vi "Least Pth Norm IIR Filter Design.vi"() -> ()   [LabVIEW 2023]
doc: "Demonstrates how to use the DFD Least Pth Norm Design VI to design advanced infinite impulse response (IIR) filters. You can learn how to configure the controls to obtain the ideal frequency response of the filter you want to design.\n\nComplete the following steps to use this VI.\n1) Run the VI.\n2) Select one example filter in the <B>Examples</B> list. This VI provides pre-defined filter specifications for each example filter.\n3) View the <B>Specifications</B> page to study the corresponding settings that describe the ideal frequency response.\n4) Observe the magnitude response and the pole-zero plot to view the characteristics of the designed filter.\n5) Click the <B>STOP</B> button to stop this VI."
uses:
  <vilib>/addons/Digital Filter Design/_Objects.llb/DFD Pole-Zero Plot.ctl
  <vilib>/addons/Digital Filter Design/_LpNorm.llb/dfd_Lp Norm Filter Type.ctl
  <vilib>/addons/Digital Filter Design/_Objects.llb/DFD Filter Obj.ctl
  <vilib>/addons/Digital Filter Design/_Objects.llb/DFD Filter Coef.ctl
  <vilib>/addons/Digital Filter Design/_Objects.llb/DFD Filter Structure Type Selector.ctl
  <vilib>/addons/Digital Filter Design/_Objects.llb/dfd_Internal Quantization Settings.ctl
  <vilib>/addons/Digital Filter Design/_Objects.llb/dfd_Internal Quantization Srcs.ctl
  <vilib>/addons/Digital Filter Design/_Objects.llb/DFD Coef Norm Type.ctl
  <vilib>/addons/Digital Filter Design/_Objects.llb/DFD Phase Setting.ctl
  <vilib>/addons/Digital Filter Design/Design.llb/DFD Least Pth Norm Design by IRLS.vi
  <vilib>/addons/Digital Filter Design/Analysis.llb/DFD Plot Freq Response (Linear-Spaced).vi
  <vilib>/addons/Digital Filter Design/NI_DigFilterLicensed.lvlib
panel:
  in  "filter out":T1={"mSRate_Fs"=1.0, "mSRate_Version"="1.0", "mSRate_Comments"="", "mSRate_OrgCoef"={"type"=enum."Undefined", "gain"=1.0, "coef a (k)"=[], "coef b (v)"=[]}, "mSRate_CurCoef"={"type"=enum."Undefined", "gain"=1.0, "coef a (k)"=[], "coef b (v)"=[]}, "mSRate_Quantized?"=FALSE, "mSRate_QCoef"={"type"=enum."Undefined", "gain"=1.0, "coef a (k)"=[], "coef b (v)"=[]}, "mSRate_QSettings"=[], "mSRate_Order"=0, "mSRate_Scaling"={"mSRate_ScaleByPowerOf2?"=FALSE, "mSRate_ScaleType"=enum."No Norm"}} {"mSRate_QSettings"."source" items=["Coef a/k"=0, "Coef b/v"=7, "Input"=1, "Output"=2, "Multiplicand"=3, "Product"=4, "Sum"=5, "Delay"=6, "Gain"=8]}
  out "Status Str":string="Idle"
  out "Status LED":bool
  in  "Graph":T7(tab)
  in  "dB on?":bool=TRUE
  out "Magnitude Response":cluster{"f0":dbl, "df":dbl, "values":dbl[]}[](graph)
  in  "phase view":T8
  out "Phase Response":cluster{"f0":dbl, "df":dbl, "values":dbl[]}[](graph)
  out "Group Delay":cluster{"f0":dbl, "df":dbl, "values":dbl[]}[](graph)
  out "Z-Plane":T9
  in  "stop":bool
  in  "Selector":enum32{"Examples", "Specifications"}(tab)
  out "Description":string
  in  "Example List":i32(listbox)
  in  "Apply":bool
  in  "p":i32=128
  in  "Group Delay":dbl=5.0
  in  "Band Specifications":T10(array[cluster])=[{"frequency point"=[{"frequency"=0.0, "magnitude"=1.0, "weight"=1.0, "phase"=0.0}, {"frequency"=0.2, "magnitude"=1.0, "weight"=1.0, "phase"=0.0}]}, {"frequency point"=[{"frequency"=0.3, "magnitude"=0.0, "weight"=1.0, "phase"=0.0}, {"frequency"=0.5, "magnitude"=0.0, "weight"=1.0, "phase"=0.0}]}] {"frequency point"."weight" format="%.2f"}
  in  "Pole Radius Constraint":dbl=0.99 min=0.0
  in  "Sampling Frequency [Hz]":dbl=1.0 format="%.2f"
  in  "Order":cluster{"numerator":i32, "denominator":i32}={"numerator"=5, "denominator"=5}
  in  "Filter Type":T11
  # "Select Help>>Show Context Help and move the cursor over the VI icon for more information."
  # "freq"
  # "magnitude"
  # "weight"
  # "phase"
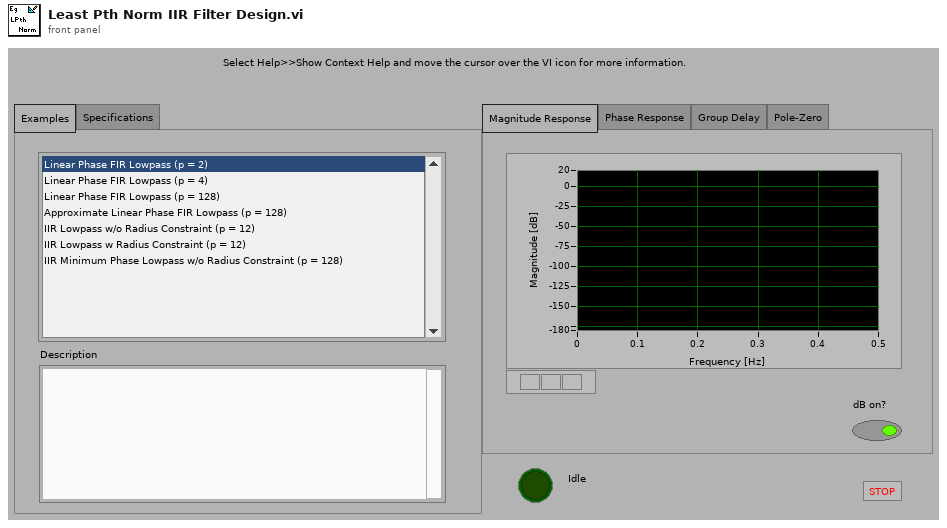
[diagram p1: front panel]
types:
  T1 = typedef "NI_DigFilterLicensed.lvlib/DFD Filter Obj.ctl" = cluster{"mSRate_Fs":dbl, "mSRate_Version":string, "mSRate_Comments":string, "mSRate_OrgCoef":T2, "mSRate_CurCoef":T2, "mSRate_Quantized?":bool, "mSRate_QCoef":T2, "mSRate_QSettings":T4[], "mSRate_Order":i32, "mSRate_Scaling":cluster{"mSRate_ScaleByPowerOf2?":bool, "mSRate_ScaleType":T6}}
  T2 = typedef "NI_DigFilterLicensed.lvlib/DFD Filter Coef.ctl" = cluster{"type":T3, "gain":dbl, "coef a (k)":dbl[], "coef b (v)":dbl[]}
  T3 = typedef "NI_DigFilterLicensed.lvlib/DFD Filter Structure Type Selector.ctl" = enum16{"Undefined", "FIR Direct Form", "FIR Direct Form Transposed", "FIR Symmetric", "FIR Antisymmetric", "IIR Direct Form I", "IIR Direct Form I Transposed", "IIR Direct Form II", "IIR Direct Form II Transposed", "IIR Cascaded Second Order Sections Form I", "IIR Cascaded Second Order Sections Form I Transposed", "IIR Cascaded Second Order Sections Form II", "IIR Cascaded Second Order Sections Form II Transposed", "Lattice Allpass (basic sections)", "Lattice Allpass (one multiplier sections)", "Lattice Allpass (normalized sections)", "Lattice AR (basic sections)", "Lattice AR (one multiplier sections)", "Lattice AR (normalized sections)", "Lattice MA (minimum phase)", "Lattice MA (maximum phase)", "Lattice ARMA (basic sections)", "Lattice ARMA (one multiplier sections)", "Lattice ARMA (normalized sections)"}
  T4 = typedef "NI_DigFilterLicensed.lvlib/dfd_Internal Quantization Settings.ctl" = cluster{"source":T5, "wl":i16, "iwl":i16, "overflow mode":enum16{"Saturation", "Wrap"}, "rounding mode":enum16{"Nearest", "Truncation"}, "signed?":bool}
  T5 = typedef "NI_DigFilterLicensed.lvlib/dfd_Internal Quantization Srcs.ctl" = u16
  T6 = typedef "NI_DigFilterLicensed.lvlib/DFD Coef Norm Type.ctl" = enum16{"No Norm", "Time Domain 1-Norm", "Time Domain 2-Norm", "Time Domain Inf-Norm"}
  T7 = enum32{"Magnitude Response", "Phase Response", "Group Delay", "Pole-Zero"}
  T8 = typedef "NI_DigFilterLicensed.lvlib/DFD Phase Setting.ctl" = cluster{"unwrap? (F)":bool, "degree? (F)":bool}
  T9 = typedef "NI_DigFilterLicensed.lvlib/DFD Pole-Zero Plot.ctl" = cluster{dbl[], dbl[]}[]
  T10 = cluster{"frequency point":cluster{"frequency":dbl, "magnitude":dbl, "weight":dbl, "phase":dbl}[]}[]
  T11 = typedef "NI_DigFilterLicensed.lvlib/dfd_Lp Norm Filter Type.ctl" = enum16{"Symmetric", "Antisymmetric", "Differentiator", "Hilbert", "Minimum Phase", "Maximum Phase"}
  T12 = cluster{"pole radius constraint":dbl, "filter type":T11, "order":cluster{"num":i32, "den":i32}, "band specs":cluster{"frequency point":cluster{"frequency":dbl, "magnitude":dbl, "weight":dbl, "phase":dbl}[]}[], "group delay":dbl, "fs [Hz]":dbl, "p (128) 2":i32}
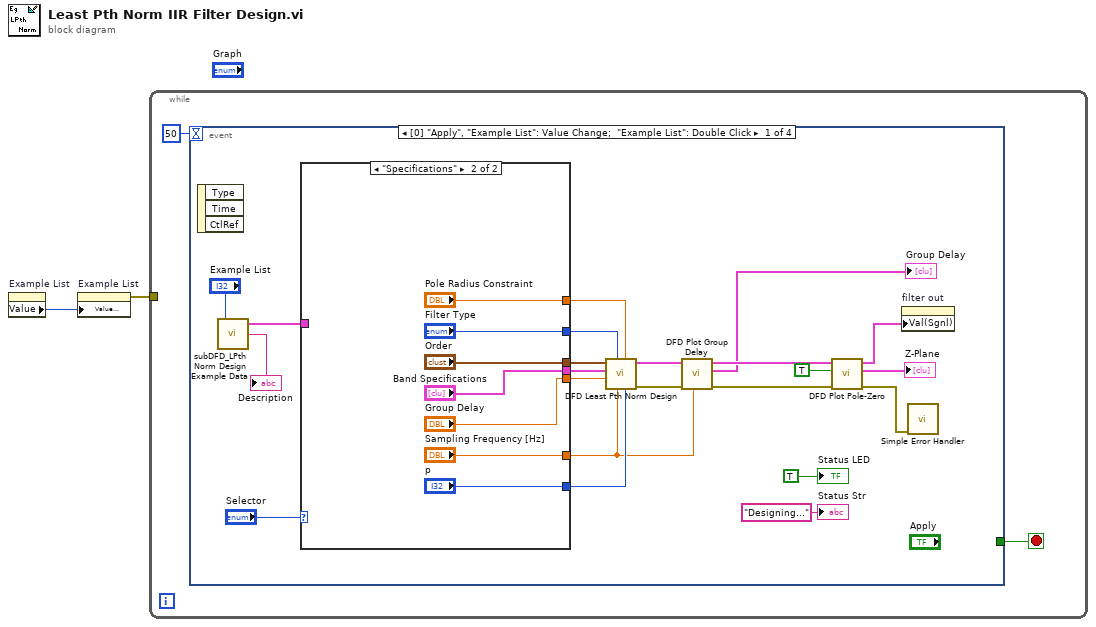
[diagram p0: block diagram]
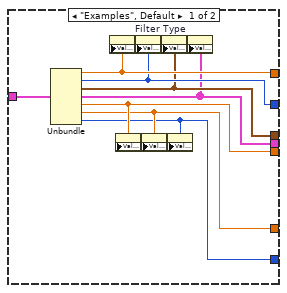
[diagram p2: hidden frame]
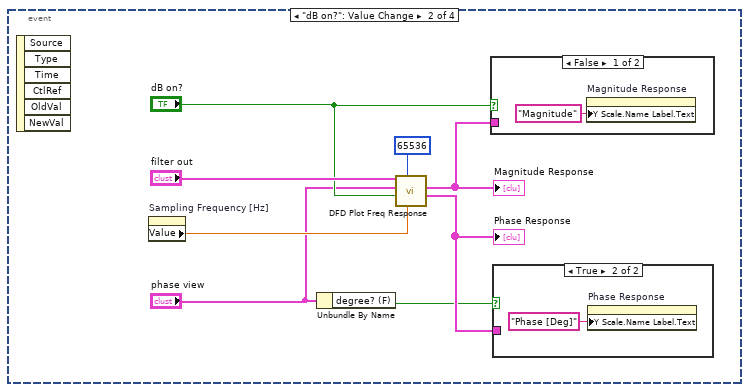
[diagram p3: hidden frame]
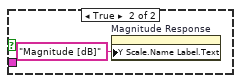
[diagram p4: hidden frame]
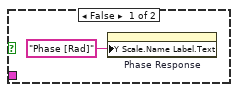
[diagram p5: hidden frame]
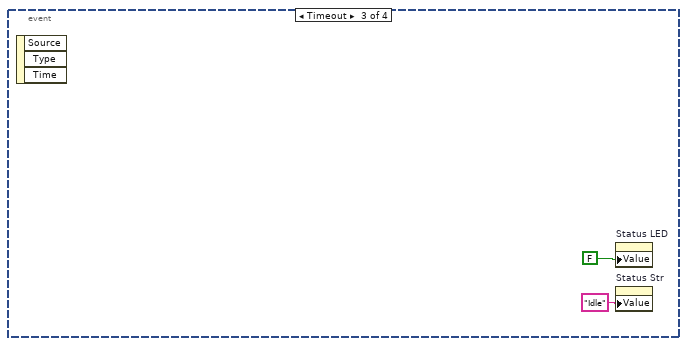
[diagram p6: hidden frame]
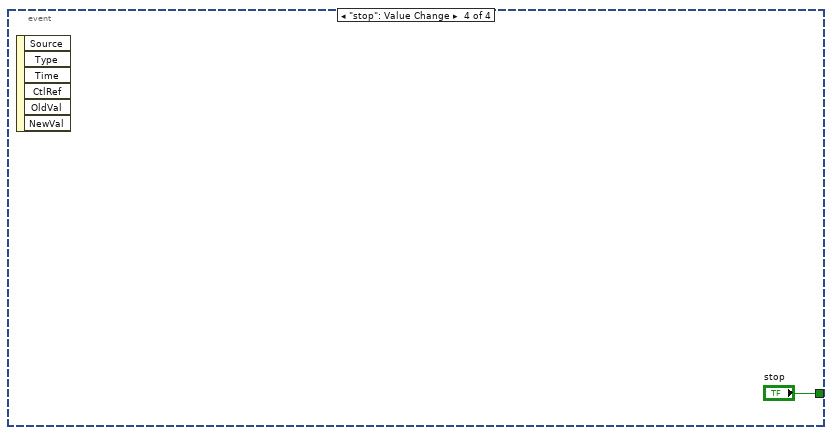
[diagram p7: hidden frame]
diagram:
  n1 = property on="Example List" class="LstBox (strict)"() -> ("Value"=w2:i32)  [unwired: 2 in, 2 out]
  n2 = property on="Example List" class="LstBox (strict)"("Value (Signaling)"=w2) -> (error out=w1:errorcluster)  [unwired: 2 in, 1 out]
  n3 = while {
    tunnel: w1 -> [_]
    stop <- w4 stop-if-true
    n4 = event shown="[0] \"Apply\", \"Example List\": Value Change;  \"Example List\": Double Click" {
      selector: _ -> [_ _ _ _]
      dyn-events: _ -> [_ _ _ _]
      timeout: 50 -> [_ _ _ _]
      tunnel: [_ _ _ "stop"] -> w4
      event "Apply", "Example List": Value Change; "Example List": Double Click {
        n5 = event-data() -> ()  [unwired: 4 out]
        n6 = call "subDFD_LPth Norm Design Example Data.vi"("Example Idx"="Example List") -> ("Spec"=w16:T12, "description"=→"Description":string)  [unwired: 1 out]
        n7 = case shown="\"Specifications\"" "Selector" {
          tunnel: [w32 "Order"] -> w23
          tunnel: [w31 "Band Specifications"] -> w22
          tunnel: [w30 "Group Delay"] -> w21
          tunnel: [w29 "Sampling Frequency [Hz]"] -> w11
          tunnel: [w28 "p"] -> w20
          tunnel: [w33 "Filter Type"] -> w19
          tunnel: [w34 "Pole Radius Constraint"] -> w18
          tunnel: w16 -> [w27 _]
          frame "Examples", Default {
            n8 = Unbundle(w27) -> ("pole radius constraint"=w34:dbl, "filter type"=w33:T11, "order"=w32:cluster{"num":i32, "den":i32}, "band specs"=w31:T10, "group delay"=w30:dbl, "fs [Hz]"=w29:dbl, "p (128) 2"=w28:i32)
            n9 = property on="Pole Radius Constraint" class="DigNum (strict)"("Value"=w34) -> ()  [unwired: 2 in, 2 out]
            n10 = property on="Group Delay" class="DigNum (strict)"("Value"=w30) -> ()  [unwired: 2 in, 2 out]
            n11 = property on="Filter Type" class="Enum (strict)"("Value"=w33) -> ()  [unwired: 2 in, 2 out]
            n12 = property on="Sampling Frequency [Hz]" class="DigNum (strict)"("Value"=w29) -> ()  [unwired: 2 in, 2 out]
            n13 = property on="Order" class="Clust (strict)"("Value"=w32) -> ()  [unwired: 2 in, 2 out]
            n14 = property on="p" class="DigNum (strict)"("Value"=w28) -> ()  [unwired: 2 in, 2 out]
            n15 = property on="Band Specifications" class="Arr (strict)"("Value"=w31) -> ()  [unwired: 2 in, 2 out]
          }
          frame "Specifications" {
          }
        }
        n16 = call-poly <vilib>:"DFD Least Pth Norm Design.vi"("p (128)"=w20, "pole radius constraint"=w18, "fs [Hz]"=w11, "filter type"=w19, "group delay"=w21, "band specs"=w22, "order"=w23) -> ("error out"=w6:errorcluster, "filter out"=w7:T1)  [unwired: 1 in, 2 out]
        n17 = call <vilib>:"DFD Plot Group Delay.vi"("fs [Hz]"=w11, "error in (no error)"=w6, "filter in"=w7) -> ("error out"=w9:errorcluster, "group delay"=→"Group Delay":cluster{"f0":dbl, "df":dbl, "values":dbl[]}[], "filter out"=w10:T1)  [unwired: 1 in, 5 out]
        n18 = call <vilib>:"DFD Plot Pole-Zero.vi"("error in (no error)"=w9, "upper half plane only"=TRUE, "filter in"=w10) -> ("error out"=w24:errorcluster, "Z-Plane"=→"Z-Plane":T9, "filter out"=w5:T1)  [unwired: 6 out]
        n19 = property on="filter out" class="Clust (strict)"("Val(Sgnl)"=w5) -> ()  [unwired: 2 in, 2 out]
        n20 = call <vilib>:"Simple Error Handler.vi"("error in (no error)"=w24) -> ()  [unwired: 1 in, 8 out]
        "Status LED" <- TRUE ("Status")
        "Status Str" <- "Designing..." ("String")
      }
      event "dB on?": Value Change {
        n21 = event-data() -> ()  [unwired: 7 out]
        n22 = property on="Sampling Frequency [Hz]" class="DigNum (strict)"() -> ("Value"=w47:dbl)  [unwired: 2 in, 2 out]
        n23 = Unbundle By Name("phase view") -> ("degree? (F)"=w42:bool)
        n24 = call-poly <vilib>:"DFD Plot Freq Response.vi"("fs [Hz]"=w47, "# freq bins"=65536 ("# freq bins (auto)"), "dB on? (T)"="dB on?", "phase view"="phase view", "filter in"="filter out") -> ("phase response"=w44:cluster{"f0":dbl, "df":dbl, "values":dbl[]}[], "magnitude response"=w45:cluster{"f0":dbl, "df":dbl, "values":dbl[]}[])  [unwired: 3 in, 2 out]
        "Magnitude Response" <- w45
        "Phase Response" <- w44
        n25 = case shown="False" "dB on?" {
          tunnel: w45 -> [_ _]
          frame False {
            n26 = property on="Magnitude Response" class="WFGraph (strict)"("Y Scale.Name Label.Text"="Magnitude") -> ()  [unwired: 2 in, 2 out]
          }
          frame True {
            n27 = property on="Magnitude Response" class="WFGraph (strict)"("Y Scale.Name Label.Text"="Magnitude [dB]") -> ()  [unwired: 2 in, 2 out]
          }
        }
        n28 = case shown="True" w42 {
          tunnel: w44 -> [_ _]
          frame False {
            n29 = property on="Phase Response" class="WFGraph (strict)"("Y Scale.Name Label.Text"="Phase [Rad]") -> ()  [unwired: 2 in, 2 out]
          }
          frame True {
            n30 = property on="Phase Response" class="WFGraph (strict)"("Y Scale.Name Label.Text"="Phase [Deg]") -> ()  [unwired: 2 in, 2 out]
          }
        }
      }
      event Timeout {
        n31 = event-data() -> ()  [unwired: 4 out]
        n32 = property on="Status LED" class="Bool (strict)"("Value"=FALSE ("Status")) -> ()  [unwired: 2 in, 2 out]
        n33 = property on="Status Str" class="Str"("Value"="Idle" ("Status")) -> ()  [unwired: 2 in, 2 out]
      }
      event "stop": Value Change {
        n34 = event-data() -> ()  [unwired: 7 out]
      }
    }
  }
